vi "CreateFilePath.vi"(8 "error in (no error)":errorcluster, 9 "data group":string, 11 "data":variant) -> (0 "error out":errorcluster, 3 "appended path":path)   [LabVIEW 2017, in "FileManager.lvlib"]
uses:
  <vilib>/addons/InsightCM/Devices/Shared/Common/FileManager/FileManager.lvlib
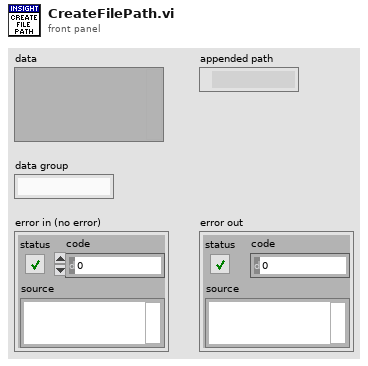
[diagram p1: front panel]
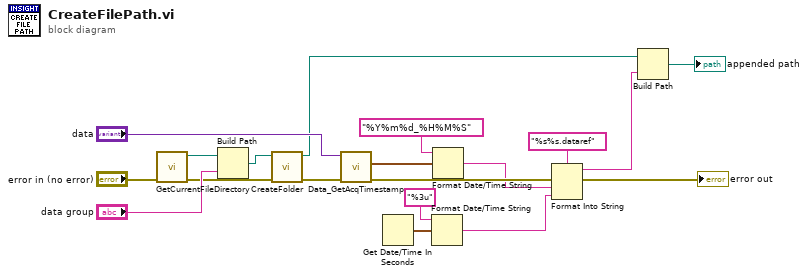
[diagram p0: block diagram]
diagram:
  n1 = call <vilib>:"GetCurrentFileDirectory.vi"("error in (no error)"="error in (no error)") -> ("error out"=w15:errorcluster, "directory"=w17:path)  [unwired: 9 in]
  n2 = Build Path(base path=w17, name or relative path="data group") -> (appended path=w11:path)
  n3 = call <vilib>:"CreateFolder.vi"("error in (no error)"=w15, "folder"=w11) -> ("error out"=w9:errorcluster, "folder out"=w12:path)  [unwired: 8 in]
  n4 = call <vilib>:"Data_GetAcqTimestamp.vi"("error in (no error)"=w9, "data"="data") -> ("error out"=w5:errorcluster, "timestamp"=w18:timestamp)  [unwired: 6 in, 2 out]
  n5 = Get Date/Time In Seconds() -> (seconds since 1Jan1904=w8:timestamp)
  n6 = Format Date/Time String(time format string (%c)="%3u", seconds (now)=w8) -> (date/time string=w2:string)  [unwired: 1 in]
  n7 = Format Date/Time String(time format string (%c)="%Y%m%d_%H%M%S", seconds (now)=w18) -> (date/time string=w3:string)  [unwired: 1 in]
  n8 = Format Into String(format string="%s%s.dataref", error in=w5, w3, w2) -> (resulting string=w1:string, error out=→"error out":errorcluster)  [unwired: 1 in]
  n9 = Build Path(base path=w12, name or relative path=w1) -> (appended path=→"appended path":path)
